vi "FPGA Main_2Modules.vi"() -> ()   [LabVIEW 2015]
doc: "This FPGA Main VI contains a control loop running in parallel with an RT watchdog loop.\n- The Control Loop performs control calculations on four input channels in parallel, and outputs the results to four output channels.\n- The RT Watchdog Loop checks for a periodic 'pet' from the RT Main VI to ensure communications between RT and FPGA are maintained."
uses:
  <vilib>/eio/EIONode/EIONode.xnode
  <vilib>/rvi/eio/common/nirviEmuTemplateMethod_errors.vi
  <vilib>/eio/EIOPropertyNode/EIOPropertyNode.xnode
  <vilib>/rvi/DataTransferAndStorage/Container/XNode/niFpgaContainer.xnode
  <vilib>/rvi/eio/common/nirviEmuTemplatePropertyGet_errors.vi
  <vilib>/rvi/eio/common/nirviEmuTemplatePropertyGet_noerrors.vi
  <vilib>/rvi/eio/common/nirviEmuTemplatePropertySet_errors.vi
  <vilib>/rvi/eio/common/nirviEmuTemplatePropertySet_noerrors.vi
  <vilib>/rvi/interface/RandomDataEmulation/nirviRandomDataFpgaReadWriteTemplate.vi
  <vilib>/LabVIEW Targets/FPGA/cRIO/shared/nicrio_ModuleControls/nicrio_cRIO-9234_DataRatesRing2.ctl
panel:
  in  "Data Rate":T1=1 items=["51.200 kS/s (NI 9234)"=1, "25.600 kS/s (NI 9234)"=2, "17.067 kS/s (NI 9234)"=3, "12.800 kS/s (NI 9234)"=4, "10.240 kS/s (NI 9234)"=5, "8.533 kS/s (NI 9234)"=6, "7.314 kS/s (NI 9234)"=7, "6.400 kS/s (NI 9234)"=8, "5.689 kS/s (NI 9234)"=9, "5.120 kS/s (NI 9234)"=10, "4.654 kS/s (NI 9234)"=11, "4.267 kS/s (NI 9234)"=12, "3.938 kS/s (NI 9234)"=13, "3.657 kS/s (NI 9234)"=14, "3.413 kS/s (NI 9234)"=15, "3.200 kS/s (NI 9234)"=16, "3.012 kS/s (NI 9234)"=17, "2.845 kS/s (NI 9234)"=18, "2.695 kS/s (NI 9234)"=19, "2.560 kS/s (NI 9234)"=20, "2.438 kS/s (NI 9234)"=21, "2.328 kS/s (NI 9234)"=22, "2.226 kS/s (NI 9234)"=23, "2.133 kS/s (NI 9234)"=24, "2.048 kS/s (NI 9234)"=25, "1.969 kS/s (NI 9234)"=26, "1.896 kS/s (NI 9234)"=27, "1.829 kS/s (NI 9234)"=28, "1.765 kS/s (NI 9234)"=29, "1.707 kS/s (NI 9234)"=30, "1.652 kS/s (NI 9234)"=31]
  out "FPGA Error":errorcluster
  out "Finished":bool
  in  "Stop":bool
  out "Module Underflow":bool
  out "DMA FIFO Full":bool
  out "Different Channel Count":bool
  out "Actual Loop Period (ticks)":u32
  out "First Read":bool
  in  "Number of Channels":i32=8
  in  "Channel Scale Array":fxp<+,24,12>[](array[numeric])=[0.0, 0.0, 0.0, 0.0, 0.0, 0.0, 0.0, 0.0]
  # "General Settings"
  # "Monitoring Values"
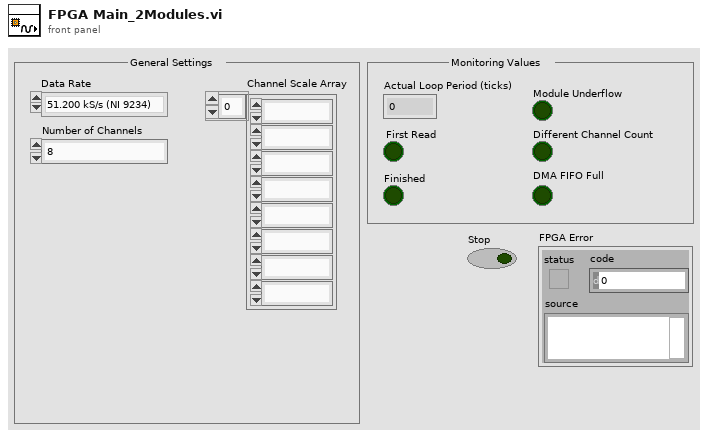
[diagram p1: front panel]
types:
  T1 = typedef "nicrio_cRIO-9234_DataRatesRing2.ctl" = u8
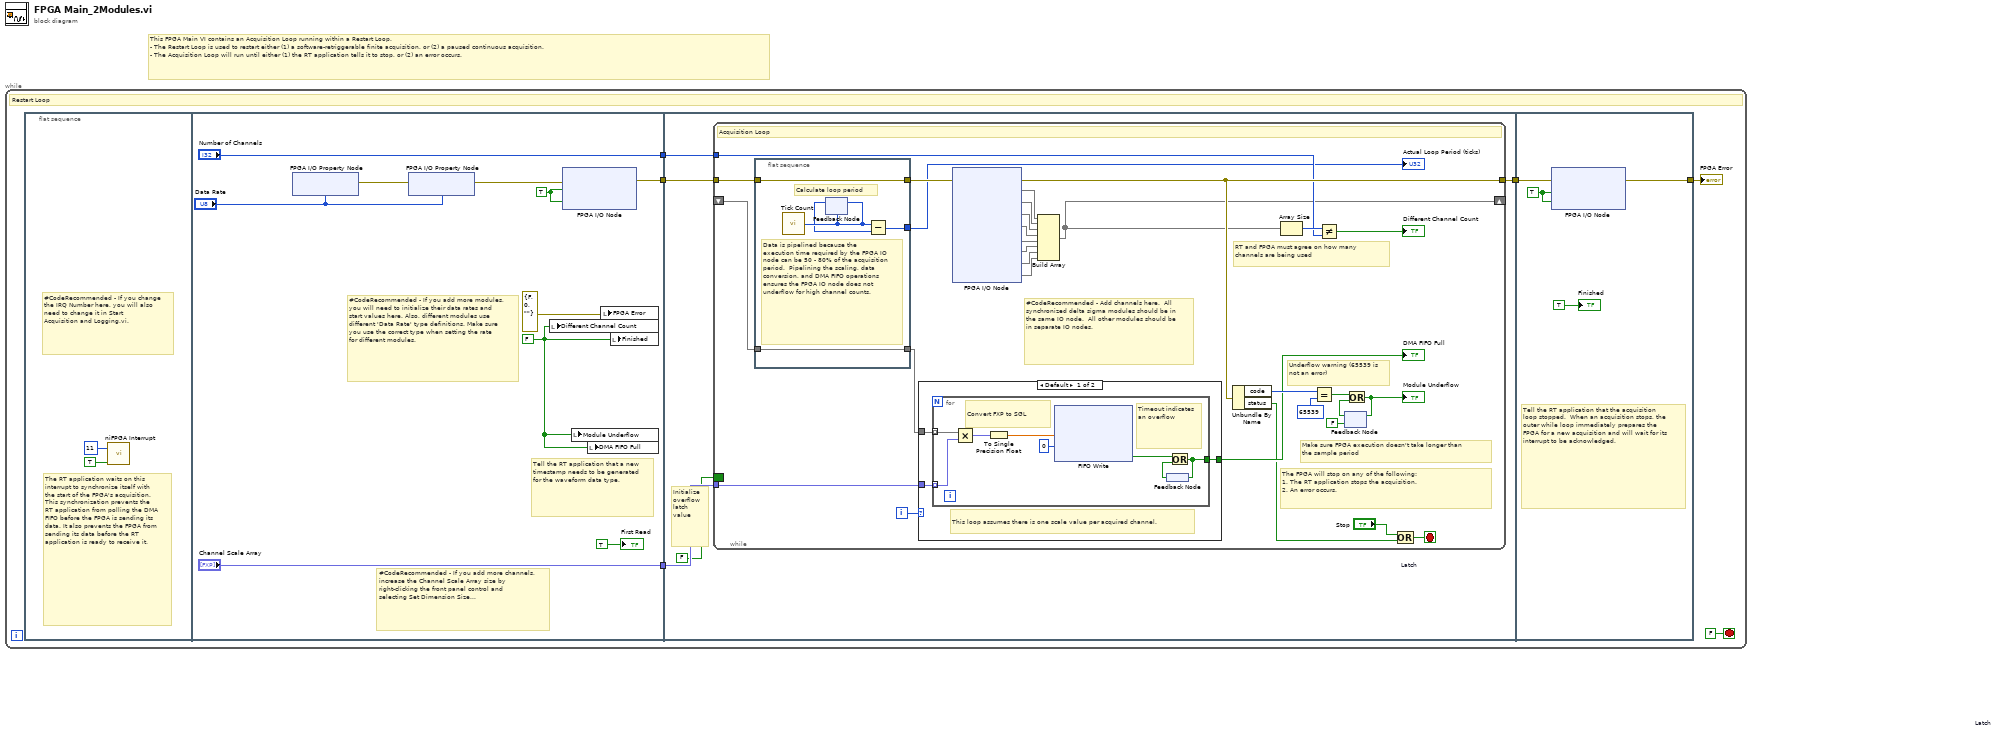
[diagram p0: block diagram]
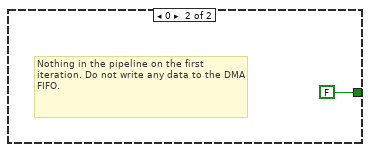
[diagram p2: hidden frame]
diagram:
  # "This FPGA Main VI contains an Acquisition Loop running within a Restart Loop.\n- The Restart Loop is used to restart either (1) a software-retriggerable finite acquisition, or (2) a paused continuous acquisition.\n- The Acquisition Loop will run until either (1) the RT application tells it to stop, or (2) an error occurs."
  n1 = while {
    stop <- FALSE stop-if-true
    # "Restart Loop"
    n2 = flat-sequence {
      tunnel: [w18] -> w5
      tunnel: ["Channel Scale Array"] -> w4
      tunnel: ["Number of Channels"] -> w3
      tunnel: w5 -> [w22]
      tunnel: w4 -> [w21]
      tunnel: w3 -> [w23]
      tunnel: [w20] -> w2
      tunnel: w2 -> [w73]
      tunnel: [w72] -> w1
      frame #0 {
        # "#CodeRecommended - If you change the IRQ Number here, you will also need to change it in Start Acquisition and Logging.vi."
        # "The RT application waits on this interrupt to synchronize itself with the start of the FPGA's acquisition.  This synchronization prevents the RT application from polling the DMA FIFO before the FPGA is sending its data. It also prevents the FPGA from sending its data before the RT application is ready to receive it."
        n3 = call <vilib>:"niFPGA Interrupt.vi"("Wait Until Cleared (F)"=TRUE ("Wait Until Cleared"), "IRQ Number (0)"=u8 11 ("IRQ Number")) -> ()  [unwired: 1 in]
      }
      frame #1 {
        w16 = FALSE ("Module Underflow")
        w11 = TRUE ("Mod1/Start")
        # "Tell the RT application that a new timestamp needs to be generated for the waveform data type."
        # "#CodeRecommended - If you add more channels, increase the Channel Scale Array size by right-clicking the front panel control and selecting Set Dimension Size..."
        # "#CodeRecommended - If you add more modules, you will need to initialize their data rates and start values here. Also, different modules use different 'Data Rate' type definitions. Make sure you use the correct type when setting the rate for different modules."
        n4 = xnode "FPGA I/O Property Node"("Data Rate"="Data Rate") -> ("error out"=w10:errorcluster)  [unwired: 2 in, 1 out]
        n5 = xnode "FPGA I/O Property Node"("error in"=w10, "Data Rate"="Data Rate") -> ("error out"=w9:errorcluster)  [unwired: 1 in, 1 out]
        n6 = local write "Different Channel Count"(w16) -> ()
        n7 = xnode "FPGA I/O Node"("error in"=w9, "Mod1/Start"=w11, "Mod2/Start"=w11) -> ("error out"=w18:errorcluster)  [unwired: 2 in, 2 out]
        n8 = local write "Module Underflow"(w16) -> ()
        n9 = local write "DMA FIFO Full"(w16) -> ()
        n10 = local write "FPGA Error"(errorcluster {"status"=FALSE, "code"=0, "source"=""} ("FPGA Error")) -> ()
        n11 = local write "Finished"(w16) -> ()
        "First Read" <- TRUE ("First Read")
      }
      frame #2 {
        # "Initialize overflow latch value"
        n12 = while {
          tunnel: w22 -> [w45]
          tunnel: [w50] -> w20
          shift-right: [w35] -> _
          shift-left: _ -> [w37]
          tunnel: w23 -> [w47]
          tunnel: w21 -> [w39]
          border: FALSE ("Overflow\nLatch") -> [_]
          i -> [w28]
          stop <- w53 stop-if-true
          # "Underflow warning (65539 is not an error)"
          # "The FPGA will stop on any of the following:\n1. The RT application stops the acquisition.\n2. An error occurs."
          # "#CodeRecommended - Add channels here.  All synchronized delta sigma modules should be in the same IO node.  All other modules should be in separate IO nodes."
          # "RT and FPGA must agree on how many channels are being used"
          # "Make sure FPGA execution doesn't take longer than the sample period"
          # "Acquisition Loop"
          n13 = flat-sequence {
            tunnel: [w70] -> w44
            tunnel: w45 -> [w70]
            tunnel: [w67] -> w43
            tunnel: w37 -> [w66]
            tunnel: [w66] -> w38
            frame #0 {
              # "Data is pipelined because the execution time required by the FPGA IO node can be 50 - 80% of the acquisition period.  Pipelining the scaling, data conversion, and DMA FIFO operations ensures the FPGA IO node does not underflow for high channel counts."
              # "Calculate loop period"
              n14 = call "Tick Count"() -> ("Tick Count(Ticks)"=w69:u32)
              n15 = feedback-in #1(w69) -> ()
              n16 = feedback #1(w69) -> (w68:u32)
              n17 = Subtract(x=w69, y=w68) -> (x-y=w67:u32)
            }
          }
          n18 = case shown="Default" w28 {
            tunnel: [w56 FALSE] -> w49
            tunnel: w39 -> [w55 _]
            tunnel: w38 -> [w54 _]
            frame Default {
              # "This loop assumes there is one scale value per acquired channel."
              n19 = for {
                tunnel: [w62] -> w56
                tunnel: w54 -> [w60] mode=indexing
                tunnel: w55 -> [w59] mode=indexing
                # "Timeout indicates an overflow"
                # "Convert FXP to SGL"
                n20 = Multiply(x=w60, y=w59) -> (x*y=w58:fxp<+,48,24>)
                n21 = To Single Precision Float(number=w58) -> (single precision float=w57:sgl)
                n22 = xnode ("FIFO Write")("Element"=w57, "Timeout"=0) -> ("Timed Out?"=w64:bool)  [unwired: 1 in, 1 out]
                n23 = feedback #2 "Latch"() -> (w63:bool)
                n24 = Or(x=w64, y=w63) -> (x .or. y?=w62:bool)
                n25 = feedback-in #2(w62) -> ()
              }
            }
            frame 0 {
              # "Nothing in the pipeline on the first iteration. Do not write any data to the DMA FIFO."
            }
          }
          "DMA FIFO Full" <- w49
          n26 = xnode "FPGA I/O Node"("error in"=w44) -> ("error out"=w50:errorcluster, "Mod1/AI0"=w42, "Mod1/AI1"=w36, "Mod1/AI2"=w41, "Mod1/AI3"=w40, "Mod2/AI0"=w27, "Mod2/AI1"=w26, "Mod2/AI2"=w25, "Mod2/AI3"=w24)  [unwired: 8 in, 8 out]
          n27 = Build Array(w42, w36, w41, w40, w27, w26, w25, w24) -> (w35:void[])
          n28 = Unbundle By Name(w50) -> ("code"=w51:i32, "status"=w30:bool)
          n29 = Array Size(array=w35) -> (size(s)=w48:i32)
          n30 = Equal?(x=w51, y=65539) -> (x = y?=w32:bool)
          n31 = Not Equal?(x=w48, y=w47) -> (x != y?=→"Different Channel Count":bool)
          n32 = feedback #3 "Latch"(FALSE) -> (w34:bool)
          n33 = Or(x=w32, y=w34) -> (x .or. y?=w31:bool)
          "Module Underflow" <- w31
          n34 = feedback-in #3(w31) -> ()
          n35 = Compound Arithmetic op=OR("Stop", w30) -> (w53:bool)
          "Actual Loop Period (ticks)" <- w43
        }
      }
      frame #3 {
        w71 = TRUE ("Mod1/Stop")
        # "Tell the RT application that the acquisition loop stopped.  When an acquisition stops, the outer while loop immediately prepares the FPGA for a new acquisition and will wait for its interrupt to be acknowledged."
        n36 = xnode "FPGA I/O Node"("error in"=w73, "Mod1/Stop"=w71, "Mod2/Stop"=w71) -> ("error out"=w72:errorcluster)  [unwired: 2 in, 2 out]
        "Finished" <- TRUE ("Finished")
      }
    }
    "FPGA Error" <- w1
  }
